vi "Main Panel.vi"() -> ()   [LabVIEW 2015]
uses:
  <vilib>/LabVIEW Interface for Arduino/Type Defs/Connection Type.ctl
  <vilib>/LabVIEW Interface for Arduino/Type Defs/Pin Mode.ctl
  <vilib>/LabVIEW Interface for Arduino/LabVIEW Interface for Arduino.lvlib
panel:
  in  "X":bool
  in  "Y":bool
  out "Shut Down":bool
  out "Battery Temperature":dbl(slide) scale=0.0..100.0
  out "Trigger Previous":dbl
  out "Trigger Feedback":dbl(knob) scale=0.0..180.0
  out "Pin4":dbl
  out "Pin2":dbl
  in  "Y Control":u8(knob)=15 scale=0.0..90.0
  in  "X Control":u8(knob)=15 scale=0.0..180.0
  out "2":dbl(slide)
  out "?":dbl(slide)
  out "Battery Voltage":dbl(knob) scale=0.0..10.0
  out "LOW BAT":bool
  out "Trigger Angle":dbl(knob) scale=0.0..180.0
  out "Right":bool
  out "Left":bool
  out "Backward":bool
  out "Forward":bool
  in  "stop":bool
  out "Manual Speed":dbl(knob) scale=0.0..255.0
  # "CONTROL BASE"
  # "MOBILE ROBOT"
  # "Robot Direction"
  # "X Control"
  # "Y Control"
  # "Servo Feedback"
  # "Battery Voltage"
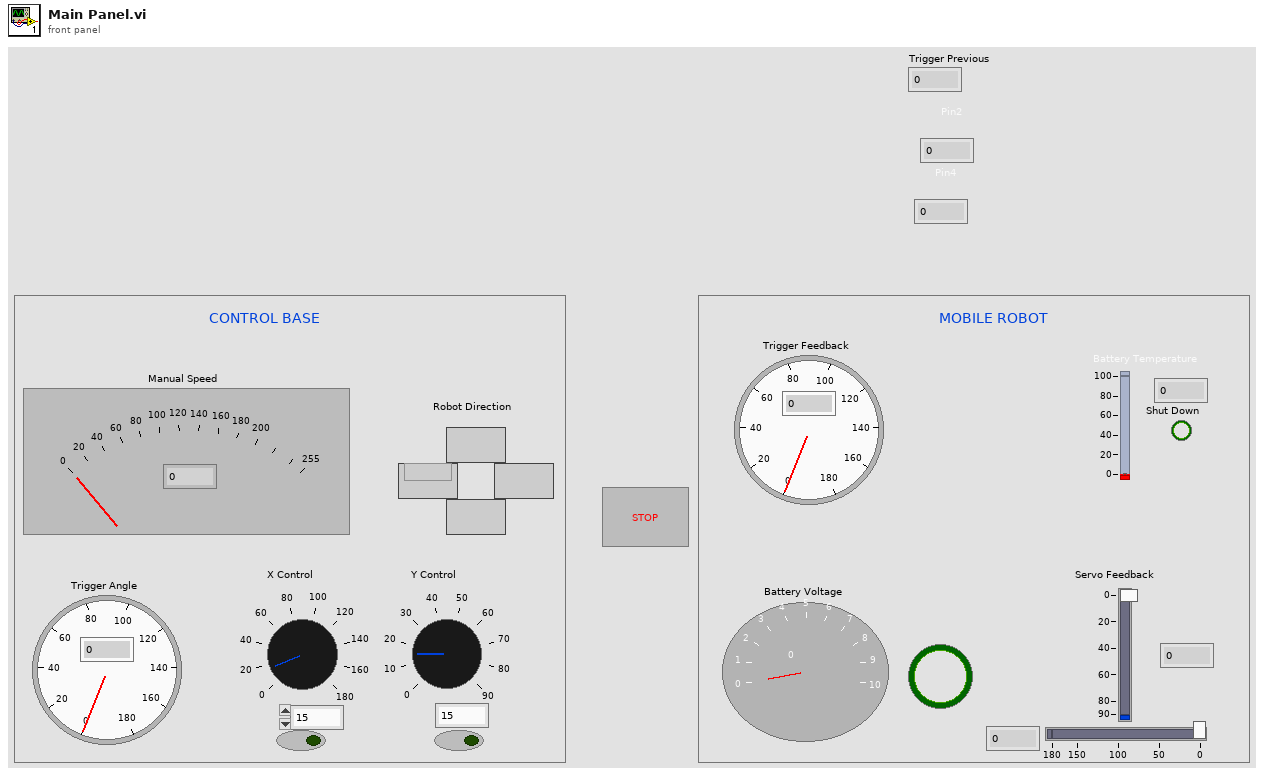
[diagram p1: front panel]
types:
  T1 = typedef "LabVIEW Interface for Arduino.lvlib/Pin Mode.ctl" = enum8{"Input", "Output"}
  T2 = typedef "LabVIEW Interface for Arduino.lvlib/Connection Type.ctl" = enum8{"USB / Serial", "XBEE", "BlueSmirf (Bluetooth)"}
  T3 = typedef "LabVIEW Interface for Arduino.lvlib/Arduino Resource.ctl" = cluster{"VISA resource":refnum<visa-resource-name>, "Board Type":T4, "Connection Type":enum8{"USB / Serial"}, "Bytes Per Packet (15)":u8}
  T4 = typedef "LabVIEW Interface for Arduino.lvlib/Board Type.ctl" = enum16{"Uno", "Dimuelanove w/Atmega 328", "Mega 2560"}
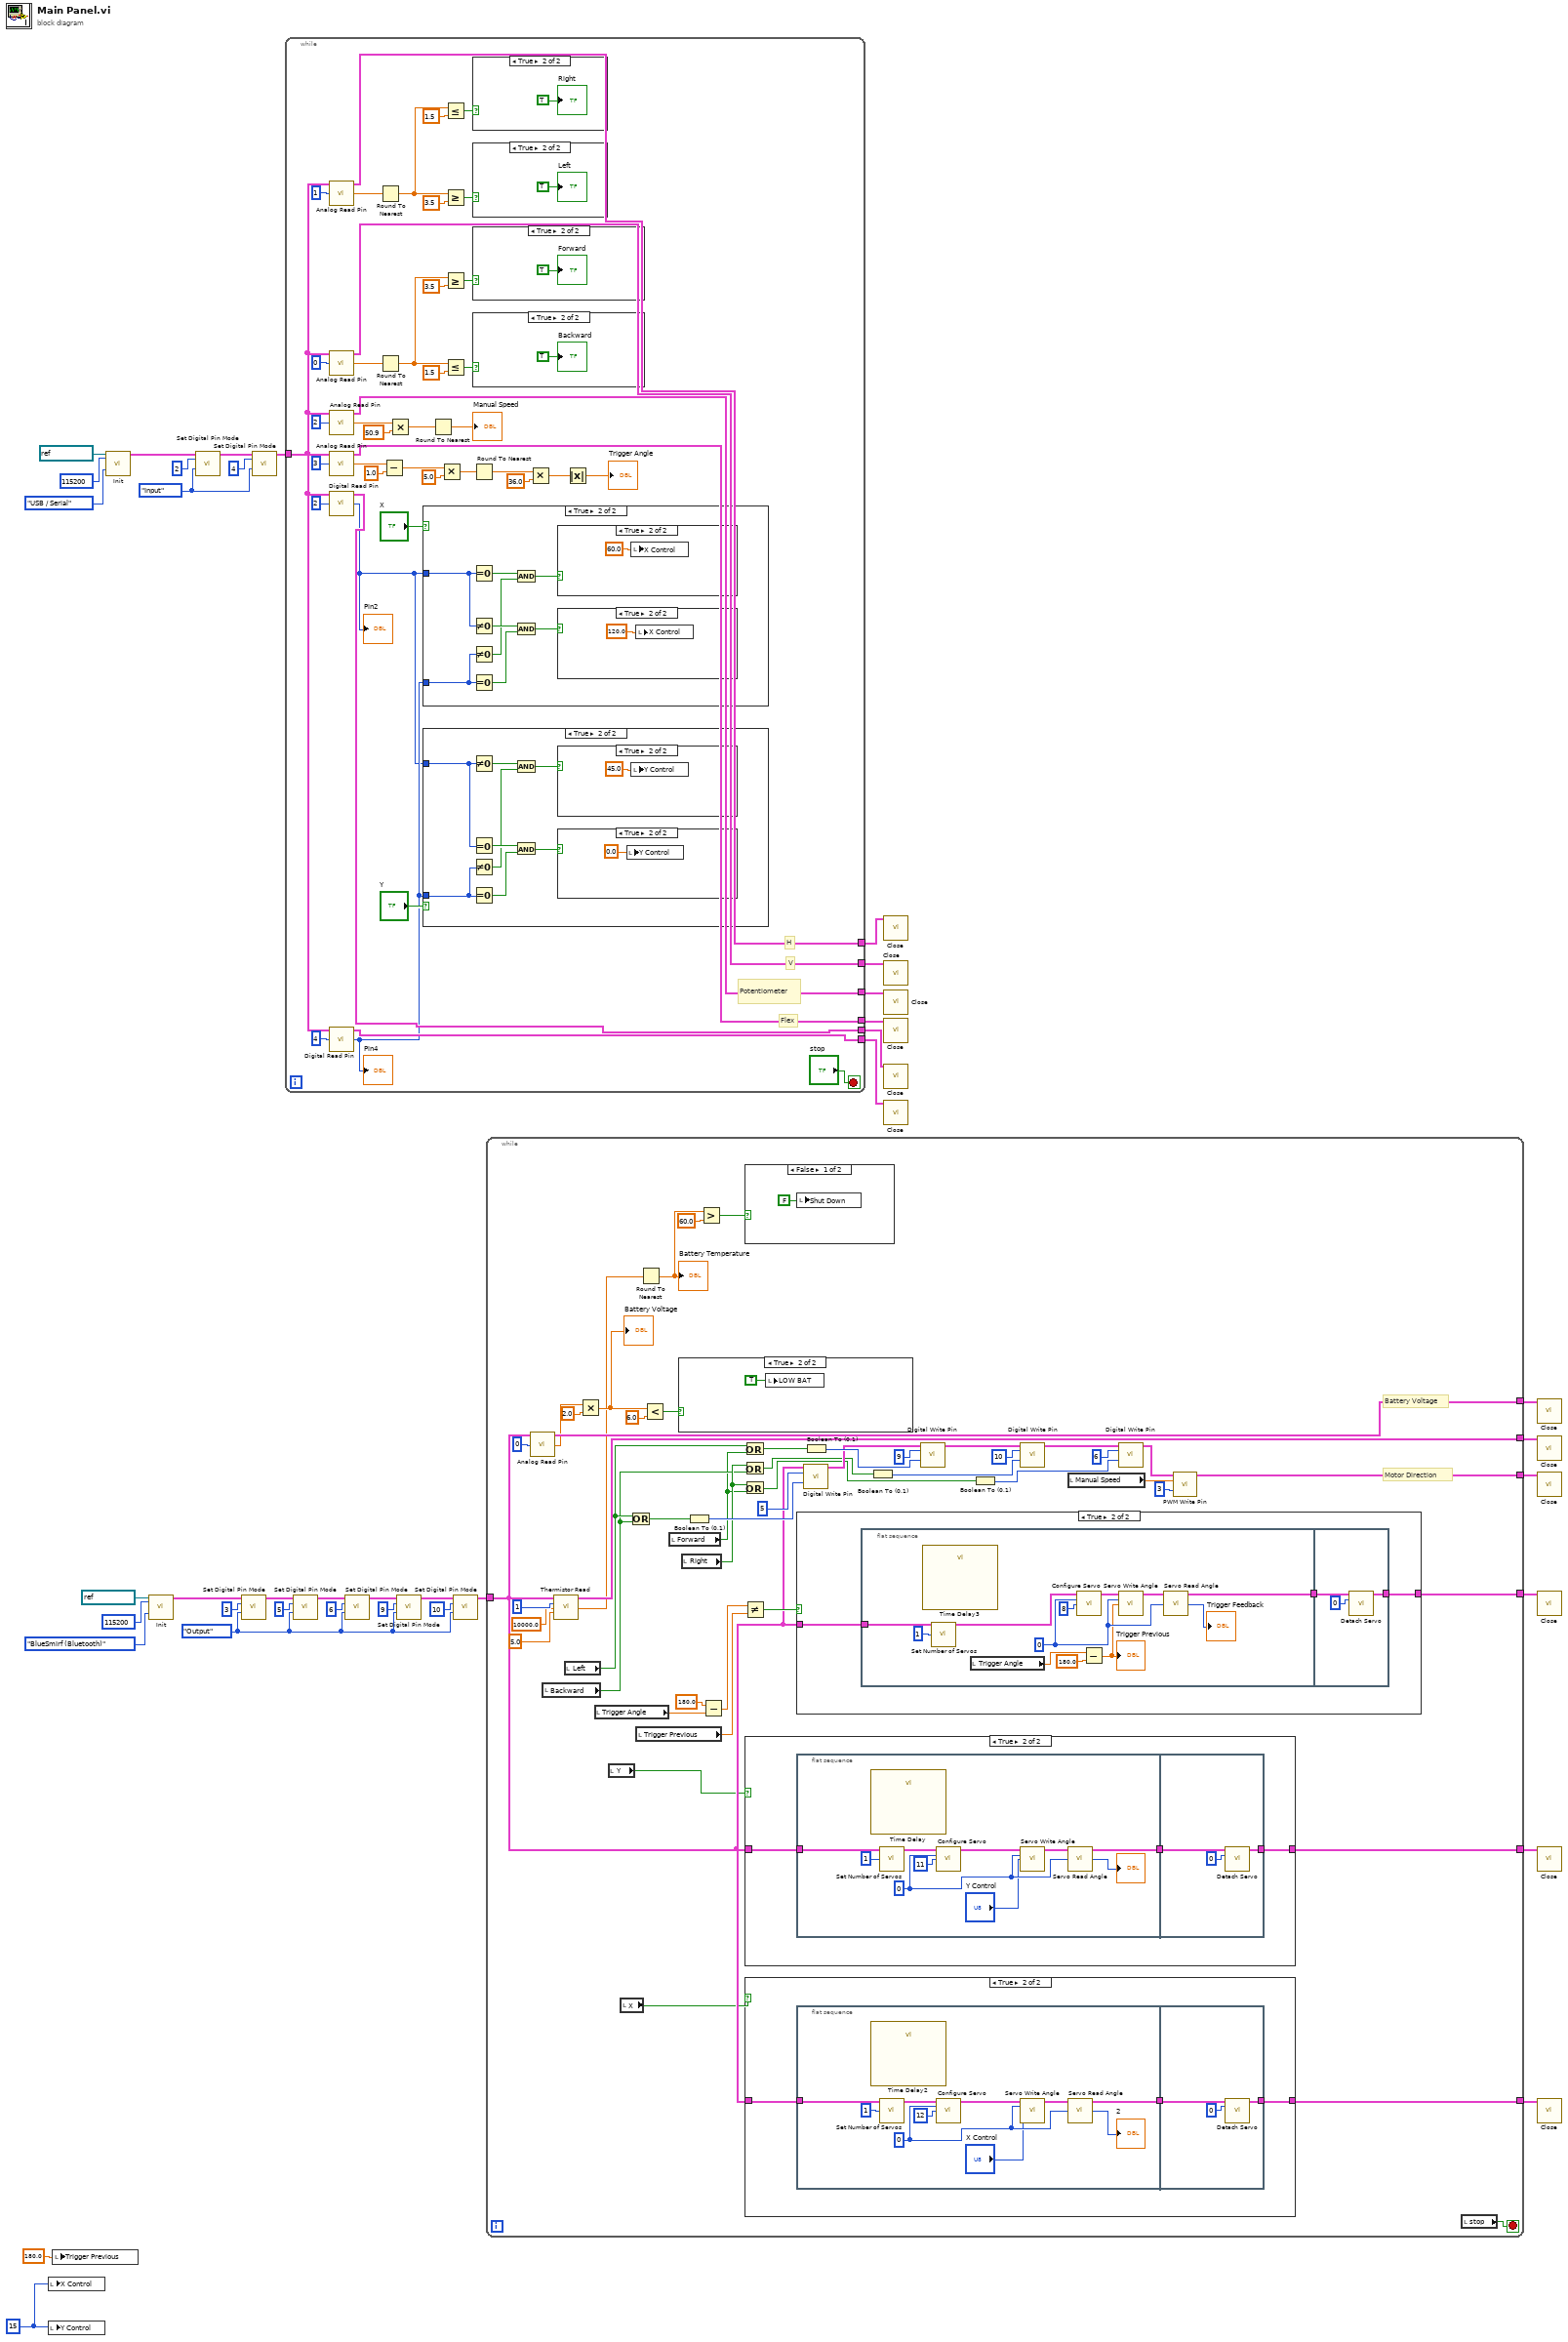
[diagram p0: block diagram]
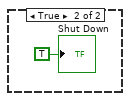
[diagram p2: hidden frame]
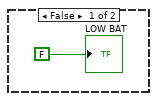
[diagram p6: hidden frame]
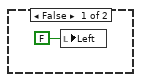
[diagram p13: hidden frame]
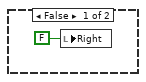
[diagram p14: hidden frame]
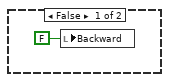
[diagram p15: hidden frame]
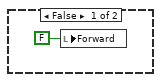
[diagram p16: hidden frame]
diagram:
  w7 = Pin_Mode."Input" ("Pin Mode (Input)")
  w1 = u8 15 ("X Control")
  w16 = Pin_Mode."Output" ("Pin Mode (Input)")
  n1 = local write "X Control"(w1) -> ()
  n2 = local write "Y Control"(w1) -> ()
  n3 = local write "Trigger Previous"(180.0 ("Trigger Previous")) -> ()
  n4 = call <vilib>:"Init.vi"("VISA resource"=refnum<visa-resource-name> "COM10", "Baud Rate (115200)"=u32 115200, "Connection Type (USB/Serial)"=Connection_Type."USB / Serial") -> ("Arduino Resource"=w5:T3)  [unwired: 15 in, 1 out]
  n5 = call <vilib>:"Init.vi"("VISA resource"=refnum<visa-resource-name> "COM11", "Baud Rate (115200)"=u32 115200, "Connection Type (USB/Serial)"=Connection_Type."BlueSmirf (Bluetooth)") -> ("Arduino Resource"=w21:T3)  [unwired: 15 in, 1 out]
  n6 = call <vilib>:"Set Digital Pin Mode.vi"("Arduino Resource"=w5, "Digital I/O Pin"=u8 2, "Pin Mode (Input)"=w7) -> ("Arduino Resource"=w10:T3)  [unwired: 11 in, 1 out]
  n7 = call <vilib>:"Set Digital Pin Mode.vi"("Arduino Resource"=w21, "Digital I/O Pin"=u8 3, "Pin Mode (Input)"=w16) -> ("Arduino Resource"=w22:T3)  [unwired: 11 in, 1 out]
  n8 = call <vilib>:"Set Digital Pin Mode.vi"("Arduino Resource"=w10, "Digital I/O Pin"=u8 4, "Pin Mode (Input)"=w7) -> ("Arduino Resource"=w6:T3)  [unwired: 11 in, 1 out]
  n9 = while {
    tunnel: w6 -> [w43]
    tunnel: [w80] -> w35
    tunnel: [w67] -> w34
    tunnel: [w59] -> w33
    tunnel: [w53] -> w32
    tunnel: [w45] -> w12
    tunnel: [w44] -> w11
    stop <- "stop" stop-if-true
    # "Flex"
    # "H"
    # "V"
    # "Potentiometer"
    n10 = call <vilib>:"Analog Read Pin.vi"("Arduino Resource"=w43, "Analog Input Pin (0)"=u8 1) -> ("Arduino Resource"=w59:T3, "Voltage"=w61:dbl)  [unwired: 11 in, 1 out]
    n11 = call <vilib>:"Analog Read Pin.vi"("Arduino Resource"=w43, "Analog Input Pin (0)"=u8 0) -> ("Arduino Resource"=w67:T3, "Voltage"=w74:dbl)  [unwired: 11 in, 1 out]
    n12 = call <vilib>:"Analog Read Pin.vi"("Arduino Resource"=w43, "Analog Input Pin (0)"=u8 2) -> ("Arduino Resource"=w80:T3, "Voltage"=w77:dbl)  [unwired: 11 in, 1 out]
    n13 = call <vilib>:"Analog Read Pin.vi"("Arduino Resource"=w43, "Analog Input Pin (0)"=u8 3) -> ("Arduino Resource"=w53:T3, "Voltage"=w57:dbl)  [unwired: 11 in, 1 out]
    n14 = call <vilib>:"Digital Read Pin.vi"("Arduino Resource"=w43, "Digital I/O Pin (0)"=u8 2 ("Analog Input Pin (0)")) -> ("Arduino Resource"=w45:T3, "Value"=w39:u8)  [unwired: 11 in, 1 out]
    "Pin2" <- w39
    n15 = call <vilib>:"Digital Read Pin.vi"("Arduino Resource"=w43, "Digital I/O Pin (0)"=u8 4 ("Analog Input Pin (0)")) -> ("Arduino Resource"=w44:T3, "Value"=w40:u8)  [unwired: 11 in, 1 out]
    "Pin4" <- w40
    n16 = Round To Nearest(number=w61) -> (nearest integer value=w63:dbl)
    n17 = Round To Nearest(number=w74) -> (nearest integer value=w71:dbl)
    n18 = Subtract(x=w57, y=1.0) -> (x-y=w54:dbl)
    n19 = Multiply(x=w77, y=50.9) -> (x*y=w76:dbl)
    n20 = case shown="True" "X" {
      tunnel: w39 -> [_ w93]
      tunnel: w40 -> [_ w92]
      frame False {
      }
      frame True {
        n21 = Equal To 0?(x=w93) -> (x = 0?=w97:bool)
        n22 = Not Equal To 0?(x=w93) -> (x != 0?=w96:bool)
        n23 = Not Equal To 0?(x=w92) -> (x != 0?=w95:bool)
        n24 = Equal To 0?(x=w92) -> (x = 0?=w94:bool)
        n25 = And(x=w97, y=w95) -> (x .and. y?=w98:bool)
        n26 = And(x=w96, y=w94) -> (x .and. y?=w99:bool)
        n27 = case shown="True" w98 {
          frame False {
          }
          frame True {
            n28 = local write "X Control"(60.0 ("x")) -> ()
          }
        }
        n29 = case shown="True" w99 {
          frame False {
          }
          frame True {
            n30 = local write "X Control"(120.0 ("x")) -> ()
          }
        }
      }
    }
    n31 = case shown="True" "Y" {
      tunnel: w40 -> [_ w83]
      tunnel: w39 -> [_ w82]
      frame False {
      }
      frame True {
        n32 = Not Equal To 0?(x=w82) -> (x != 0?=w85:bool)
        n33 = Equal To 0?(x=w82) -> (x = 0?=w89:bool)
        n34 = Not Equal To 0?(x=w83) -> (x != 0?=w84:bool)
        n35 = Equal To 0?(x=w83) -> (x = 0?=w88:bool)
        n36 = And(x=w85, y=w84) -> (x .and. y?=w86:bool)
        n37 = And(x=w89, y=w88) -> (x .and. y?=w87:bool)
        n38 = case shown="True" w86 {
          frame False {
          }
          frame True {
            n39 = local write "Y Control"(45.0 ("x")) -> ()
          }
        }
        n40 = case shown="True" w87 {
          frame False {
          }
          frame True {
            n41 = local write "Y Control"(0.0 ("x")) -> ()
          }
        }
      }
    }
    n42 = Round To Nearest(number=w76) -> (nearest integer value=→"Manual Speed":dbl)
    n43 = Multiply(x=w54, y=5.0) -> (x*y=w52:dbl)
    n44 = Less Or Equal?(x=w63, y=1.5) -> (x <= y?=w66:bool)
    n45 = Greater Or Equal?(x=w63, y=3.5) -> (x >= y?=w65:bool)
    n46 = Greater Or Equal?(x=w71, y=3.5) -> (x >= y?=w73:bool)
    n47 = Less Or Equal?(x=w71, y=1.5) -> (x <= y?=w70:bool)
    n48 = Round To Nearest(number=w52) -> (nearest integer value=w50:dbl)
    n49 = case shown="True" w66 {
      frame False {
        n50 = local write "Right"(FALSE ("Right")) -> ()
      }
      frame True {
        "Right" <- TRUE ("Right")
      }
    }
    n51 = case shown="True" w65 {
      frame False {
        n52 = local write "Left"(FALSE ("Right")) -> ()
      }
      frame True {
        "Left" <- TRUE ("Left")
      }
    }
    n53 = case shown="True" w73 {
      frame False {
        n54 = local write "Forward"(FALSE ("Right")) -> ()
      }
      frame True {
        "Forward" <- TRUE ("Forward")
      }
    }
    n55 = case shown="True" w70 {
      frame False {
        n56 = local write "Backward"(FALSE ("Right")) -> ()
      }
      frame True {
        "Backward" <- TRUE ("Backward")
      }
    }
    n57 = Multiply(x=w50, y=36.0) -> (x*y=w49:dbl)
    n58 = Absolute Value(x=w49) -> (abs(x)=→"Trigger Angle":dbl)
  }
  n59 = call <vilib>:"Set Digital Pin Mode.vi"("Arduino Resource"=w22, "Digital I/O Pin"=u8 5, "Pin Mode (Input)"=w16) -> ("Arduino Resource"=w23:T3)  [unwired: 11 in, 1 out]
  n60 = call <vilib>:"Set Digital Pin Mode.vi"("Arduino Resource"=w23, "Digital I/O Pin"=u8 6, "Pin Mode (Input)"=w16) -> ("Arduino Resource"=w19:T3)  [unwired: 11 in, 1 out]
  n61 = call <vilib>:"Set Digital Pin Mode.vi"("Arduino Resource"=w19, "Digital I/O Pin"=u8 9, "Pin Mode (Input)"=w16) -> ("Arduino Resource"=w17:T3)  [unwired: 11 in, 1 out]
  n62 = call <vilib>:"Set Digital Pin Mode.vi"("Arduino Resource"=w17, "Digital I/O Pin"=u8 10, "Pin Mode (Input)"=w16) -> ("Arduino Resource"=w15:T3)  [unwired: 11 in, 1 out]
  n63 = while {
    tunnel: w15 -> [w120]
    tunnel: [w158] -> w28
    tunnel: [w130] -> w27
    tunnel: [w128] -> w14
    tunnel: [w127] -> w13
    tunnel: [w121] -> w3
    tunnel: [w116] -> w2
    stop <- w159 stop-if-true
    # "Battery Voltage"
    # "Motor Direction"
    n64 = call <vilib>:"Analog Read Pin.vi"("Arduino Resource"=w120, "Analog Input Pin (0)"=u8 0) -> ("Arduino Resource"=w158:T3, "Voltage"=w156:dbl)  [unwired: 11 in, 1 out]
    n65 = local read "Backward"() -> (w132:bool)
    n66 = call <vilib>:"Thermistor Read.vi"("Arduino Resource"=w120, "Thermistor AI Pin (0)"=u8 1, "Paired Resistance (10K Ohms)"=10000.0, "Vcc (5 v)"=5.0) -> ("Arduino Resource"=w116:T3, "Temperature"=w115:dbl)  [unwired: 9 in, 1 out]
    n67 = local read "Left"() -> (w137:bool)
    n68 = Multiply(x=w156, y=2.0) -> (x*y=w129:dbl)
    "Battery Voltage" <- w129
    n69 = local read "Trigger Angle"() -> (w122:dbl)
    n70 = local read "Y"() -> (w111:bool)
    n71 = local read "X"() -> (w110:bool)
    n72 = Or(x=w137, y=w132) -> (x .or. y?=w138:bool)
    n73 = local read "Trigger Previous"() -> (w124:dbl)
    n74 = Round To Nearest(number=w115) -> (nearest integer value=w114:dbl)
    "Battery Temperature" <- w114
    n75 = Less?(x=w129, y=6.0) -> (x < y?=w153:bool)
    n76 = local read "Forward"() -> (w131:bool)
    n77 = case shown="True" w153 {
      frame False {
        "LOW BAT" <- FALSE ("Right")
      }
      frame True {
        n78 = local write "LOW BAT"(TRUE ("Left")) -> ()
      }
    }
    n79 = local read "Right"() -> (w134:bool)
    n80 = Boolean To (0,1)(Boolean=w138) -> (0, 1=w151:i16)
    n81 = Greater?(x=w114, y=60.0) -> (0:w112:bool)
    n82 = Subtract(x=180.0 ("y"), y=w122) -> (x-y=w126:dbl)
    n83 = Or(x=w137, y=w131) -> (x .or. y?=w136:bool)
    n84 = Or(x=w134, y=w132) -> (x .or. y?=w133:bool)
    n85 = Or(x=w134, y=w131) -> (x .or. y?=w135:bool)
    n86 = Not Equal?(x=w126, y=w124) -> (x != y?=w125:bool)
    n87 = case shown="False" w112 {
      frame False {
        n88 = local write "Shut Down"(FALSE ("Shut Down")) -> ()
      }
      frame True {
        "Shut Down" <- TRUE ("Shut Down")
      }
    }
    n89 = case shown="True" w111 {
      tunnel: w120 -> [w198 w201]
      tunnel: [w198 w199] -> w128
      frame False {
      }
      frame True {
        n90 = flat-sequence {
          tunnel: w201 -> [w211]
          tunnel: [w205] -> w200
          tunnel: w200 -> [w213]
          tunnel: [w212] -> w199
          frame #0 {
            w204 = u8 0 ("Servo Number (0)")
            n91 = call "Time Delay"() -> ()  [unwired: 11 in, 1 out]
            n92 = call <vilib>:"Set Number of Servos.vi"("Arduino Resource"=w211, "Number Of Servos (1)"=u8 1) -> ("Arduino Resource"=w208:T3)  [unwired: 12 in, 1 out]
            n93 = call <vilib>:"Configure Servo.vi"("Arduino Resource"=w208, "Servo Number (0)"=w204, "DIO Pin (2)"=u8 11) -> ("Arduino Resource"=w207:T3)  [unwired: 11 in, 1 out]
            n94 = call <vilib>:"Servo Write Angle.vi"("Arduino Resource"=w207, "Servo Number"=w204, "Angle (Degrees)"="Y Control") -> ("Arduino Resource"=w206:T3)  [unwired: 11 in, 1 out]
            n95 = call <vilib>:"Servo Read Angle.vi"("Arduino Resource"=w206, "Servo Number"=w204) -> ("Arduino Resource"=w205:T3, "Angle (Degrees)"=→"?":u8)  [unwired: 11 in, 1 out]
          }
          frame #1 {
            n96 = call <vilib>:"Detach Servo.vi"("Arduino Resource"=w213, "Servo Number"=u8 0) -> ("Arduino Resource"=w212:T3)  [unwired: 12 in, 1 out]
          }
        }
      }
    }
    n97 = case shown="True" w110 {
      tunnel: [w181 w182] -> w127
      tunnel: w120 -> [w181 w184]
      frame False {
      }
      frame True {
        n98 = flat-sequence {
          tunnel: w184 -> [w190]
          tunnel: [w188] -> w183
          tunnel: w183 -> [w196]
          tunnel: [w195] -> w182
          frame #0 {
            w187 = u8 0 ("Servo Number (0)")
            n99 = call "Time Delay2"() -> ()  [unwired: 11 in, 1 out]
            n100 = call <vilib>:"Set Number of Servos.vi"("Arduino Resource"=w190, "Number Of Servos (1)"=u8 1) -> ("Arduino Resource"=w194:T3)  [unwired: 12 in, 1 out]
            n101 = call <vilib>:"Configure Servo.vi"("Arduino Resource"=w194, "Servo Number (0)"=w187, "DIO Pin (2)"=u8 12) -> ("Arduino Resource"=w191:T3)  [unwired: 11 in, 1 out]
            n102 = call <vilib>:"Servo Write Angle.vi"("Arduino Resource"=w191, "Servo Number"=w187, "Angle (Degrees)"="X Control") -> ("Arduino Resource"=w189:T3)  [unwired: 11 in, 1 out]
            n103 = call <vilib>:"Servo Read Angle.vi"("Arduino Resource"=w189, "Servo Number"=w187) -> ("Arduino Resource"=w188:T3, "Angle (Degrees)"=→"2":u8)  [unwired: 11 in, 1 out]
          }
          frame #1 {
            n104 = call <vilib>:"Detach Servo.vi"("Arduino Resource"=w196, "Servo Number"=u8 0) -> ("Arduino Resource"=w195:T3)  [unwired: 12 in, 1 out]
          }
        }
      }
    }
    n105 = case shown="True" w125 {
      tunnel: [w162 w164] -> w121
      tunnel: w120 -> [w162 w163]
      frame False {
      }
      frame True {
        n106 = flat-sequence {
          tunnel: [w172] -> w165
          tunnel: w163 -> [w166]
          tunnel: w165 -> [w179]
          tunnel: [w178] -> w164
          frame #0 {
            w171 = u8 0 ("Servo Number (0)")
            n107 = call "Time Delay3"() -> ()  [unwired: 11 in, 1 out]
            n108 = call <vilib>:"Set Number of Servos.vi"("Arduino Resource"=w166, "Number Of Servos (1)"=u8 1) -> ("Arduino Resource"=w175:T3)  [unwired: 12 in, 1 out]
            n109 = local read "Trigger Angle"() -> (w168:dbl)
            n110 = call <vilib>:"Configure Servo.vi"("Arduino Resource"=w175, "Servo Number (0)"=w171, "DIO Pin (2)"=u8 8) -> ("Arduino Resource"=w174:T3)  [unwired: 11 in, 1 out]
            n111 = Subtract(x=w168, y=180.0) -> (x-y=w167:dbl)
            "Trigger Previous" <- w167
            n112 = call <vilib>:"Servo Write Angle.vi"("Arduino Resource"=w174, "Servo Number"=w171, "Angle (Degrees)"=w167) -> ("Arduino Resource"=w173:T3)  [unwired: 11 in, 1 out]
            n113 = call <vilib>:"Servo Read Angle.vi"("Arduino Resource"=w173, "Servo Number"=w171) -> ("Arduino Resource"=w172:T3, "Angle (Degrees)"=→"Trigger Feedback":u8)  [unwired: 11 in, 1 out]
          }
          frame #1 {
            n114 = call <vilib>:"Detach Servo.vi"("Arduino Resource"=w179, "Servo Number"=u8 0) -> ("Arduino Resource"=w178:T3)  [unwired: 12 in, 1 out]
          }
        }
      }
    }
    n115 = call <vilib>:"Digital Write Pin.vi"("Arduino Resource"=w120, "Digital I/O Pin (0)"=u8 5, "Value (0)"=w151) -> ("Arduino Resource"=w144:T3)  [unwired: 11 in, 1 out]
    n116 = Boolean To (0,1)(Boolean=w136) -> (0, 1=w150:i16)
    n117 = Boolean To (0,1)(Boolean=w133) -> (0, 1=w147:i16)
    n118 = call <vilib>:"Digital Write Pin.vi"("Arduino Resource"=w144, "Digital I/O Pin (0)"=u8 9, "Value (0)"=w150) -> ("Arduino Resource"=w143:T3)  [unwired: 11 in, 1 out]
    n119 = Boolean To (0,1)(Boolean=w135) -> (0, 1=w146:i16)
    n120 = call <vilib>:"Digital Write Pin.vi"("Arduino Resource"=w143, "Digital I/O Pin (0)"=u8 10, "Value (0)"=w147) -> ("Arduino Resource"=w142:T3)  [unwired: 11 in, 1 out]
    n121 = local read "Manual Speed"() -> (w139:dbl)
    n122 = call <vilib>:"Digital Write Pin.vi"("Arduino Resource"=w142, "Digital I/O Pin (0)"=u8 6, "Value (0)"=w146) -> ("Arduino Resource"=w140:T3)  [unwired: 11 in, 1 out]
    n123 = call <vilib>:"PWM Write Pin.vi"("Arduino Resource"=w140, "Duty Cycle (0 - 255)"=w139, "PWM Pin (3)"=u8 3) -> ("Arduino Resource"=w130:T3)  [unwired: 11 in, 1 out]
    n124 = local read "stop"() -> (w159:bool)
  }
  n125 = call <vilib>:"Close.vi"("Arduino Resource"=w33) -> ()  [unwired: 14 in, 1 out]
  n126 = call <vilib>:"Close.vi"("Arduino Resource"=w34) -> ()  [unwired: 14 in, 1 out]
  n127 = call <vilib>:"Close.vi"("Arduino Resource"=w35) -> ()  [unwired: 14 in, 1 out]
  n128 = call <vilib>:"Close.vi"("Arduino Resource"=w32) -> ()  [unwired: 14 in, 1 out]
  n129 = call <vilib>:"Close.vi"("Arduino Resource"=w12) -> ()  [unwired: 14 in, 1 out]
  n130 = call <vilib>:"Close.vi"("Arduino Resource"=w11) -> ()  [unwired: 14 in, 1 out]
  n131 = call <vilib>:"Close.vi"("Arduino Resource"=w28) -> ()  [unwired: 14 in, 1 out]
  n132 = call <vilib>:"Close.vi"("Arduino Resource"=w2) -> ()  [unwired: 14 in, 1 out]
  n133 = call <vilib>:"Close.vi"("Arduino Resource"=w27) -> ()  [unwired: 14 in, 1 out]
  n134 = call <vilib>:"Close.vi"("Arduino Resource"=w3) -> ()  [unwired: 14 in, 1 out]
  n135 = call <vilib>:"Close.vi"("Arduino Resource"=w14) -> ()  [unwired: 14 in, 1 out]
  n136 = call <vilib>:"Close.vi"("Arduino Resource"=w13) -> ()  [unwired: 14 in, 1 out]
